vi "3_1_Fxp_addation.vi"(1 "y":fxp<+/-,1,3>, 2 "x":fxp<+/-,1,3>) -> (0 "x+y":fxp<+/-,2,4> format="%.41g")   [LabVIEW 2020]
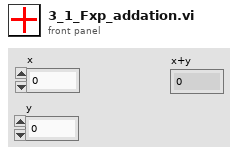
[diagram p1: front panel]
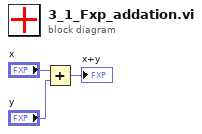
[diagram p0: block diagram]
diagram:
  n1 = Add(x="x", y="y") -> (x+y=→"x+y":fxp<+/-,2,4>)
